vi "getData.vi"(8 "error in (no error)":errorcluster, 11 "Record in":refnum<class "Record.lvclass">) -> (0 "error out":errorcluster, 3 "Record out":refnum<class "Record.lvclass">)   [LabVIEW 2017, in "Error Log.lvlib" / "Record.lvclass"]
uses:
  Record.lvclass
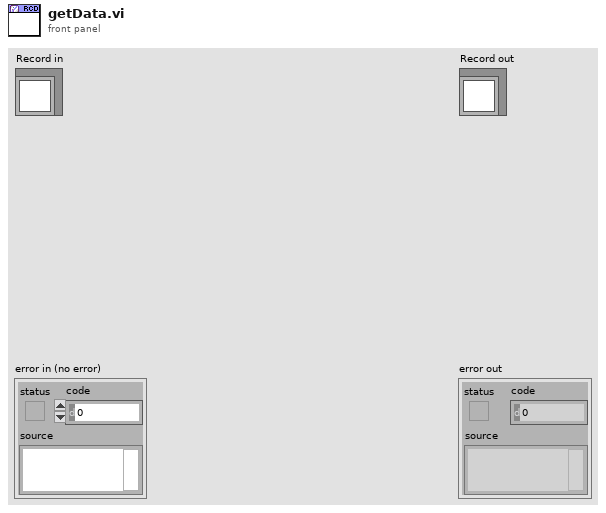
[diagram p1: front panel]
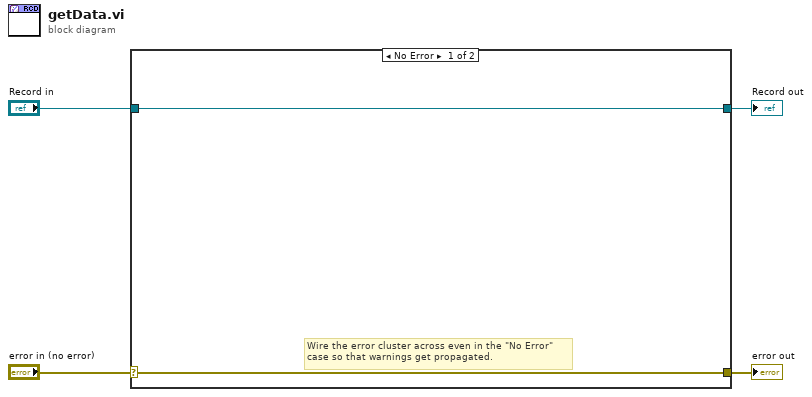
[diagram p0: block diagram]
diagram:
  n1 = case shown="No Error" "error in (no error)" {
    selector: "error in (no error)" -> [w5 w8]
    tunnel: [w5 w8] -> w3
    tunnel: [w6 w7] -> w1
    tunnel: "Record in" -> [w6 w7]
    frame No Error {
      # "Wire the error cluster across even in the \"No Error\"\ncase so that warnings get propagated."
    }
    frame Error {
    }
  }
  "error out" <- w3
  "Record out" <- w1
